vi "Sam Thermometer.vi"() -> ()   [LabVIEW 2013]
panel:
  in  "System on/off":bool
  out "Air Conditioning":bool
  in  "Heat/Cool":bool
  out "Outside Temperature":dbl(slide) scale=0.0..100.0
  out "Furnace":bool
  in  "Emergency Stop":bool
  in  "Desired Temperature":dbl(knob) scale=0.0..100.0
  out "Thermometer":dbl(slide) scale=0.0..100.0
  # "Heat"
  # "Cool"
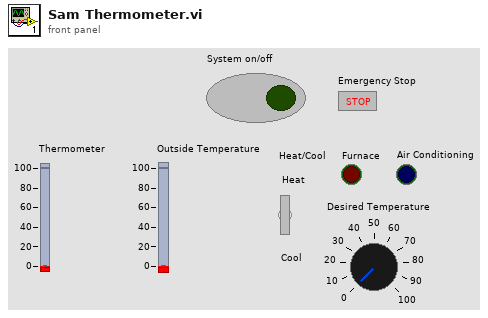
[diagram p1: front panel]
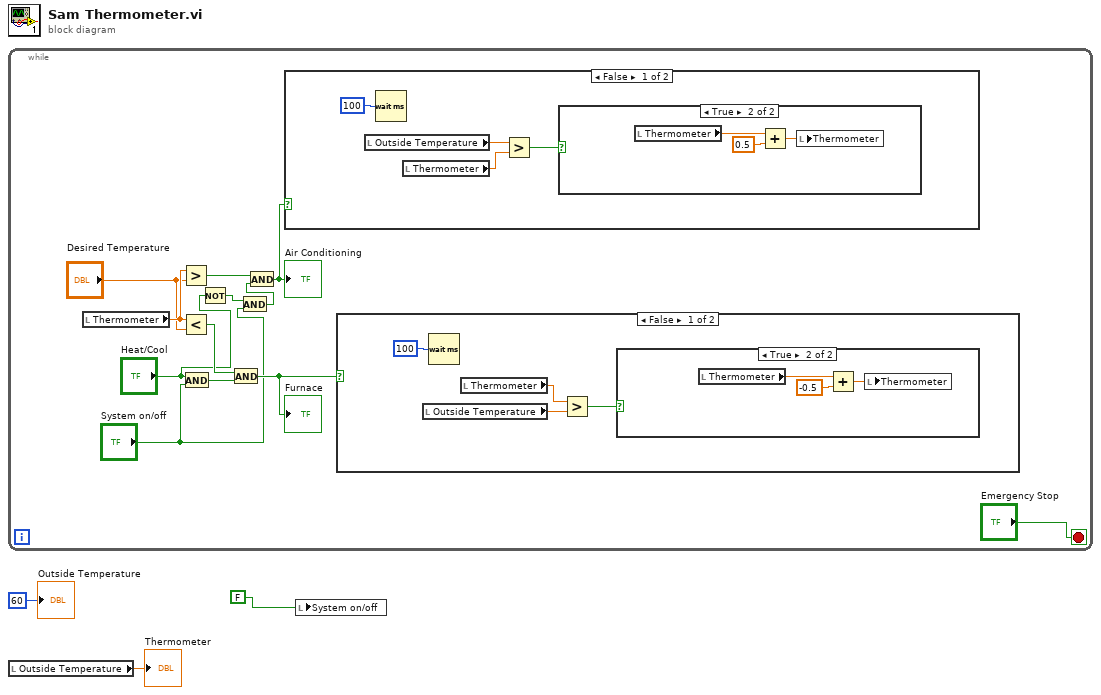
[diagram p0: block diagram]
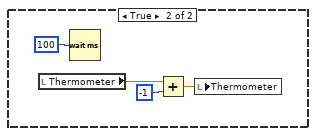
[diagram p3: hidden frame]
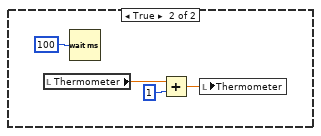
[diagram p5: hidden frame]
diagram:
  n1 = while {
    stop <- "Emergency Stop" stop-if-true
    n2 = local read "Thermometer"() -> (w14:dbl)
    n3 = Greater?(x=w14, y="Desired Temperature") -> (0:w10:bool)
    n4 = Less?(x=w14, y="Desired Temperature") -> (x < y?=w12:bool)
    n5 = And(x="Heat/Cool", y="System on/off") -> (x .and. y?=w8:bool)
    n6 = Not(x="Heat/Cool") -> (.not. x?=w6:bool)
    n7 = And(x=w12, y=w8) -> (x .and. y?=w11:bool)
    "Furnace" <- w11
    n8 = And(x=w6, y="System on/off") -> (x .and. y?=w4:bool)
    n9 = And(x=w10, y=w4) -> (x .and. y?=w9:bool)
    "Air Conditioning" <- w9
    n10 = case shown="False" w9 {
      frame False {
        n11 = local read "Outside Temperature"() -> (w18:dbl)
        n12 = Wait (ms)(milliseconds to wait=100) -> ()  [unwired: 1 out]
        n13 = local read "Thermometer"() -> (w17:dbl)
        n14 = Greater?(x=w18, y=w17) -> (0:w16:bool)
        n15 = case shown="True" w16 {
          frame False {
          }
          frame True {
            n16 = local read "Thermometer"() -> (w22:dbl)
            n17 = Add(x=w22, y=0.5) -> (x+y=w21:dbl)
            n18 = local write "Thermometer"(w21) -> ()
          }
        }
      }
      frame True {
        n19 = local read "Thermometer"() -> (w26:dbl)
        n20 = Wait (ms)(milliseconds to wait=100) -> ()  [unwired: 1 out]
        n21 = Add(x=w26, y=-1) -> (x+y=w25:dbl)
        n22 = local write "Thermometer"(w25) -> ()
      }
    }
    n23 = case shown="False" w11 {
      frame False {
        n24 = local read "Outside Temperature"() -> (w28:dbl)
        n25 = Wait (ms)(milliseconds to wait=100) -> ()  [unwired: 1 out]
        n26 = local read "Thermometer"() -> (w29:dbl)
        n27 = Greater?(x=w29, y=w28) -> (0:w27:bool)
        n28 = case shown="True" w27 {
          frame False {
          }
          frame True {
            n29 = local read "Thermometer"() -> (w33:dbl)
            n30 = Add(x=w33, y=-0.5) -> (x+y=w32:dbl)
            n31 = local write "Thermometer"(w32) -> ()
          }
        }
      }
      frame True {
        n32 = local read "Thermometer"() -> (w37:dbl)
        n33 = Wait (ms)(milliseconds to wait=100) -> ()  [unwired: 1 out]
        n34 = Add(x=w37, y=1) -> (x+y=w36:dbl)
        n35 = local write "Thermometer"(w36) -> ()
      }
    }
  }
  n36 = local read "Outside Temperature"() -> (→"Thermometer":dbl)
  n37 = local write "System on/off"(FALSE) -> ()
  "Outside Temperature" <- 60
